vi "test - Cluster.vi"(8 "error in (no error)":errorcluster, 11 "TestCase in":refnum<class "testcase-Supported-Datatype.lvclass">) -> (0 "error out":errorcluster, 3 "TestCase out":refnum<class "testcase-Supported-Datatype.lvclass">)   [LabVIEW 2017, in "testcase-Supported-Datatype.lvclass"]
uses:
  testcase-Supported-Datatype.lvclass
  6f388fa7-7212-46fd-8b74-19af36b6ef65.vi
  addons/API-String-Arugments-Support/_Support/Data To API String Arguments.vi
  <vilib>/addons/_JKI Toolkits/VI Tester/TestCase.llb/TestCase.lvclass
  addons/API-String-Arugments-Support/API String Arguments Support.lvlib
  C:/Program Files (x86)/National Instruments/LabVIEW 2017/vi.lib/addons/_JKI Toolkits/VI Tester/TestCase.llb/TestCase.lvclass
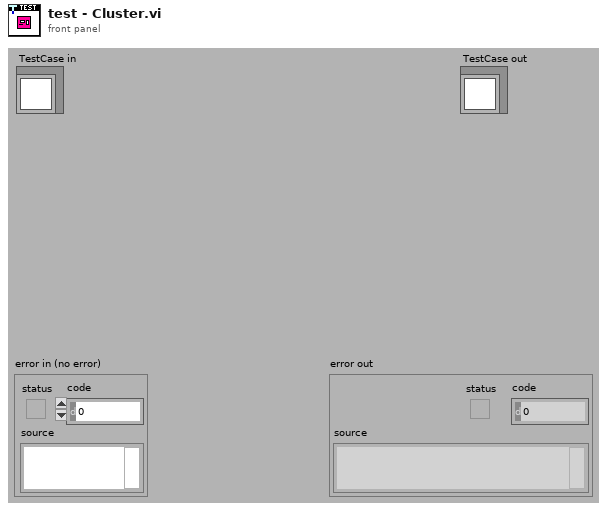
[diagram p1: front panel]
types:
  T1 = cluster{"Child":string[], "Name":string, "Bool":bool}
  T2 = cluster{"Child":cluster{"Name":string}, "Name":string, "Bool":bool}
  T3 = cluster{"Name":string, "Child":cluster{"Name":string}, "Bool":bool}
  T4 = cluster{"a":string, "xxx":cluster{"b":string, "c":string, "yyy":cluster{"d":string, "e":string}}, "zzz":cluster{"d":string, "e":string}}
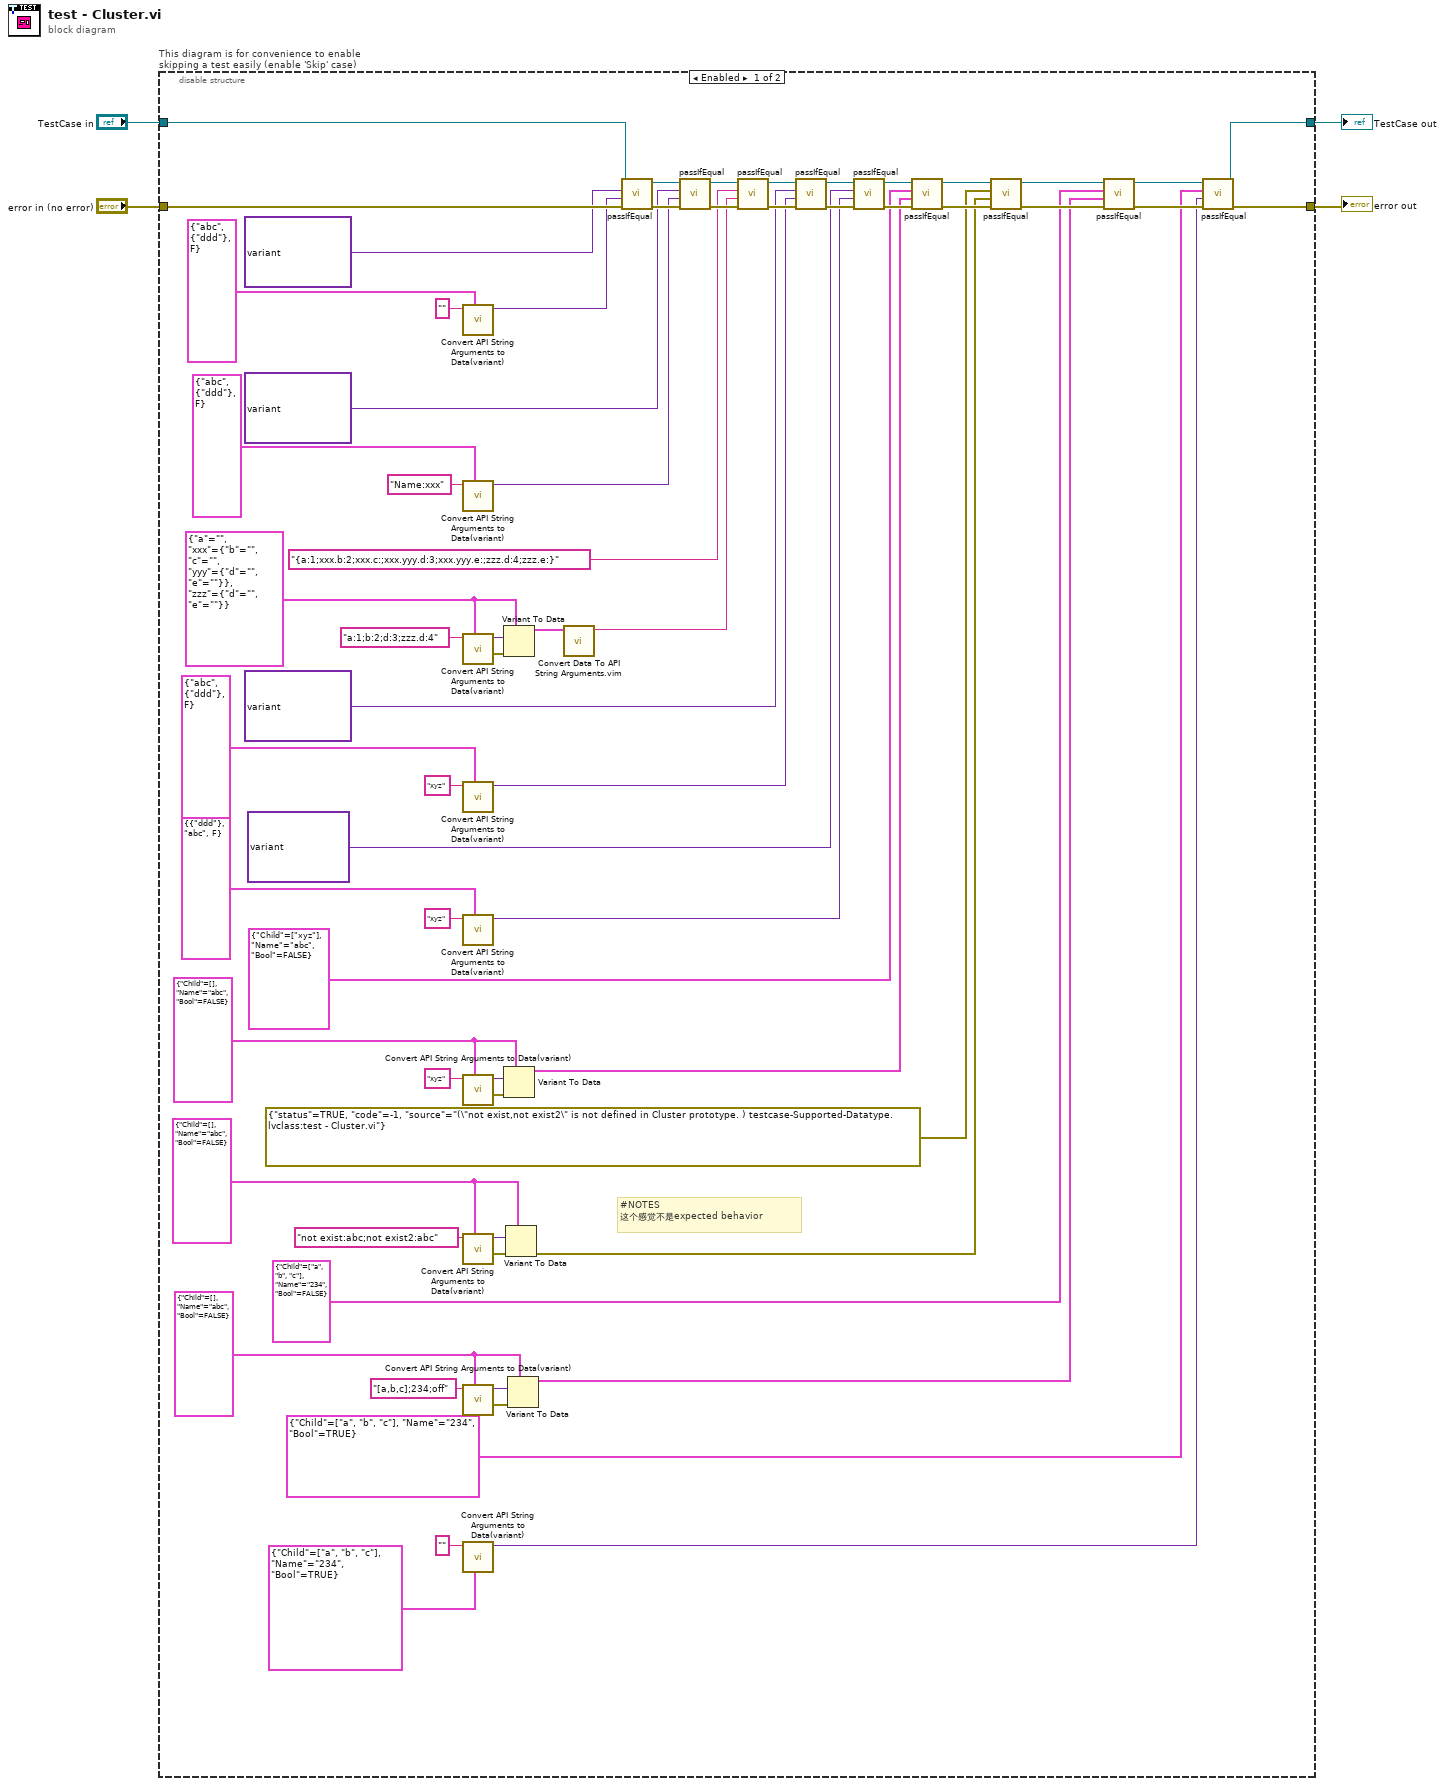
[diagram p0: block diagram]
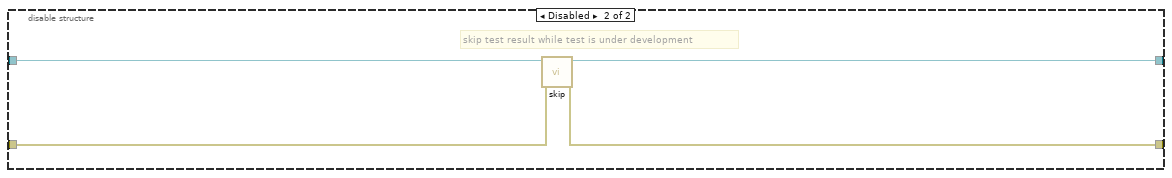
[diagram p2: hidden frame]
diagram:
  n1 = disable-structure "This diagram is for convenience to enable skipping a test easily (enable 'Skip' case)" shown="Enabled" {
    disable-tunnel: "TestCase in" -> [w69 w73]
    disable-tunnel: [w31 w71] -> w1
    disable-tunnel: [w30 w72] -> w3
    disable-tunnel: "error in (no error)" -> [w68 w70]
    frame Enabled {
      w8 = T1 {"Child"=[], "Name"="abc", "Bool"=FALSE} ("Data 8")
      w11 = T1 {"Child"=[], "Name"="abc", "Bool"=FALSE} ("Data 8")
      w13 = T1 {"Child"=[], "Name"="abc", "Bool"=FALSE} ("Data 8")
      w23 = T4 {"a"="", "xxx"={"b"="", "c"="", "yyy"={"d"="", "e"=""}}, "zzz"={"d"="", "e"=""}} ("Data 8")
      # "#NOTES\n这个感觉不是expected behavior"
      n2 = call "Convert API String Arguments to Data(variant).vi"("Type"=T3 {"Name"="abc", "Child"={"Name"="ddd"}, "Bool"=FALSE} ("Data 8"), "String"="") -> ("Data"=w27:variant)  [unwired: 8 in, 1 out]
      n3 = call "Convert API String Arguments to Data(variant).vi"("Type"=T3 {"Name"="abc", "Child"={"Name"="ddd"}, "Bool"=FALSE} ("Data 8"), "String"="Name:xxx") -> ("Data"=w25:variant)  [unwired: 8 in, 1 out]
      n4 = call "Convert API String Arguments to Data(variant).vi"("Type"=w23, "String"="a:1;b:2;d:3;zzz.d:4") -> ("error"=w61:errorcluster, "Data"=w62:variant)  [unwired: 8 in]
      n5 = call "Convert API String Arguments to Data(variant).vi"("Type"=T3 {"Name"="abc", "Child"={"Name"="ddd"}, "Bool"=FALSE} ("Data 8"), "String"="xyz") -> ("Data"=w18:variant)  [unwired: 8 in, 1 out]
      n6 = call "Convert API String Arguments to Data(variant).vi"("Type"=T2 {"Child"={"Name"="ddd"}, "Name"="abc", "Bool"=FALSE} ("Data 8"), "String"="xyz") -> ("Data"=w15:variant)  [unwired: 8 in, 1 out]
      n7 = call "Convert API String Arguments to Data(variant).vi"("Type"=w13, "String"="xyz") -> ("error"=w50:errorcluster, "Data"=w51:variant)  [unwired: 8 in]
      n8 = call "Convert API String Arguments to Data(variant).vi"("Type"=w11, "String"="not exist:abc;not exist2:abc") -> ("error"=w46:errorcluster, "Data"=w45:variant)  [unwired: 8 in]
      n9 = call "Convert API String Arguments to Data(variant).vi"("Type"=w8, "String"="[a,b,c];234;off") -> ("error"=w39:errorcluster, "Data"=w40:variant)  [unwired: 8 in]
      n10 = call "Convert API String Arguments to Data(variant).vi"("Type"=T1 {"Child"=["a", "b", "c"], "Name"="234", "Bool"=TRUE} ("Data 8"), "String"="") -> ("Data"=w32:variant)  [unwired: 8 in, 1 out]
      n11 = Variant To Data(error in=w61, type=w23, Variant=w62) -> (data=w21:T4)  [unwired: 1 out]
      n12 = Variant To Data(error in=w50, type=w13, Variant=w51) -> (data=w47:T1)  [unwired: 1 out]
      n13 = Variant To Data(error in=w46, type=w11, Variant=w45) -> (error out=w9:errorcluster)  [unwired: 1 out]
      n14 = Variant To Data(error in=w39, type=w8, Variant=w40) -> (data=w36:T1)  [unwired: 1 out]
      n15 = call "Convert Data To API String Arguments.vim"("Data"=w21) -> ("API String"=w20:string)  [unwired: 7 in, 1 out]
      n16 = call-dynamic "passIfEqual.vi"("error in (no error)"=w68, "y"=w27, "x"=variant(cluster{"Name":string, "Child":cluster{"Name":string}, "Bool":bool} {"Name"="abc", "Child"={"Name"="ddd"}, "Bool"=FALSE}) ("Data 4"), "TestCase in"=w69) -> ("error out"=w65:errorcluster, "TestCase out"=w64:refnum<class "testcase-Supported-Datatype.lvclass">)  [unwired: 6 in]
      n17 = call-dynamic "passIfEqual.vi"("error in (no error)"=w65, "y"=w25, "x"=variant(cluster{"Name":string, "Child":cluster{"Name":string}, "Bool":bool} {"Name"="xxx", "Child"={"Name"="ddd"}, "Bool"=FALSE}) ("Data 5"), "TestCase in"=w64) -> ("error out"=w60:errorcluster, "TestCase out"=w59:refnum<class "testcase-Supported-Datatype.lvclass">)  [unwired: 6 in]
      n18 = call-dynamic "passIfEqual.vi"("error in (no error)"=w60, "y"=w20, "x"="{a:1;xxx.b:2;xxx.c:;xxx.yyy.d:3;xxx.yyy.e:;zzz.d:4;zzz.e:}" ("String"), "TestCase in"=w59) -> ("error out"=w56:errorcluster, "TestCase out"=w57:refnum<class "testcase-Supported-Datatype.lvclass">)  [unwired: 6 in]
      n19 = call-dynamic "passIfEqual.vi"("error in (no error)"=w56, "y"=w18, "x"=variant(cluster{"Name":string, "Child":cluster{"Name":string}, "Bool":bool} {"Name"="xyz", "Child"={"Name"="ddd"}, "Bool"=FALSE}) ("Data 3"), "TestCase in"=w57) -> ("error out"=w54:errorcluster, "TestCase out"=w53:refnum<class "testcase-Supported-Datatype.lvclass">)  [unwired: 6 in]
      n20 = call-dynamic "passIfEqual.vi"("error in (no error)"=w54, "y"=w15, "x"=variant(cluster{"Child":cluster{"Origin Argurment String":string}, "Name":string, "Bool":bool} {"Child"={"Origin Argurment String"="xyz"}, "Name"="abc", "Bool"=FALSE}) ("Data 2"), "TestCase in"=w53) -> ("error out"=w49:errorcluster, "TestCase out"=w48:refnum<class "testcase-Supported-Datatype.lvclass">)  [unwired: 6 in]
      n21 = call-dynamic "passIfEqual.vi"("error in (no error)"=w49, "y"=w47, "x"=T1 {"Child"=["xyz"], "Name"="abc", "Bool"=FALSE} ("data 1"), "TestCase in"=w48) -> ("error out"=w42:errorcluster, "TestCase out"=w43:refnum<class "testcase-Supported-Datatype.lvclass">)  [unwired: 6 in]
      n22 = call-dynamic "passIfEqual.vi"("error in (no error)"=w42, "y"=w9, "x"=errorcluster {"status"=TRUE, "code"=-1, "source"="(\"not exist,not exist2\" is not defined in Cluster prototype. ) testcase-Supported-Datatype.lvclass:test - Cluster.vi"} ("error 6"), "TestCase in"=w43) -> ("error out"=w37:errorcluster, "TestCase out"=w38:refnum<class "testcase-Supported-Datatype.lvclass">)  [unwired: 6 in]
      n23 = call-dynamic "passIfEqual.vi"("error in (no error)"=w37, "y"=w36, "x"=T1 {"Child"=["a", "b", "c"], "Name"="234", "Bool"=FALSE} ("data 7"), "TestCase in"=w38) -> ("error out"=w33:errorcluster, "TestCase out"=w34:refnum<class "testcase-Supported-Datatype.lvclass">)  [unwired: 6 in]
      n24 = call-dynamic "passIfEqual.vi"("error in (no error)"=w33, "y"=w32, "x"=T1 {"Child"=["a", "b", "c"], "Name"="234", "Bool"=TRUE} ("data 8"), "TestCase in"=w34) -> ("error out"=w30:errorcluster, "TestCase out"=w31:refnum<class "testcase-Supported-Datatype.lvclass">)  [unwired: 6 in]
    }
    frame Disabled {
      # "skip test result while test is under development"
      n25 = call <vilib>:"skip.vi"("error in (no error)"=w70, "TestCase in"=w73) -> ("error out"=w72:errorcluster, "TestCase out"=w71:refnum<class "testcase-Supported-Datatype.lvclass">)  [unwired: 8 in]
    }
  }
  "error out" <- w3
  "TestCase out" <- w1
